vi "FTW-Time-RelativeTimer.vi"(0 "Previous Time":dbl format="%.3fmsec\n%<%D:%H:%M:%S%3u>t", 11 "error in":errorcluster) -> (4 "Current Time":dbl format="%.3fmsec\n%<%D:%H:%M:%S%3u>t", 6 "Elapsed Time":dbl format="%.4psec", 15 "error out":errorcluster)   [LabVIEW 2014]
panel:
  # "Inputs"
  # "Outputs"
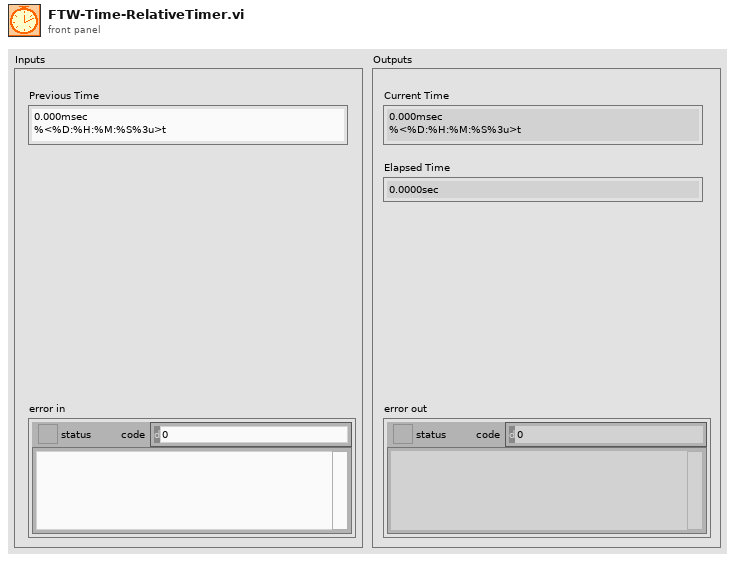
[diagram p1: front panel]
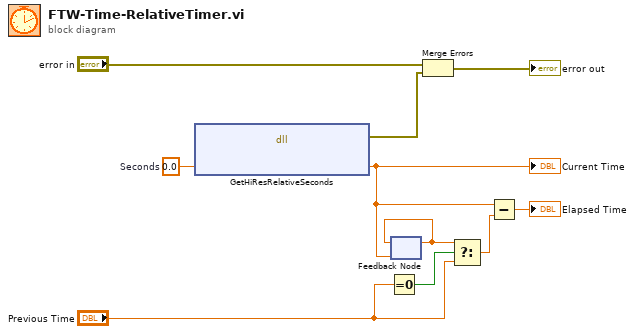
[diagram p0: block diagram]
diagram:
  w10 = 0.0  # Seconds
  n1 = dll-call lib="LabVIEW" fn="GetHiResRelativeSeconds"("Seconds"=w10) -> (error out=w3:errorcluster, "Seconds"=w7:dbl)  [unwired: 4 in, 1 out]
  "Current Time" <- w7
  n2 = Equal To 0?(x="Previous Time") -> (x = 0?=w6:bool)
  n3 = feedback #1(w7) -> (w1:dbl)
  n4 = feedback-in #1(w1) -> ()
  n5 = Merge Errors("error in", w3) -> (→"error out":errorcluster)
  n6 = Select(t=w1, s=w6, f="Previous Time") -> (s? t:f=w2:dbl)
  n7 = Subtract(x=w7, y=w2) -> (x-y=→"Elapsed Time":dbl)
